vi "Test.vi"() -> ()   [LabVIEW 2021]
panel:
  out "x-1":i32
  out "size(s)":i32[](array[numeric])
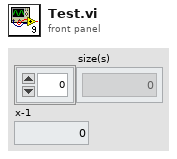
[diagram p1: front panel]
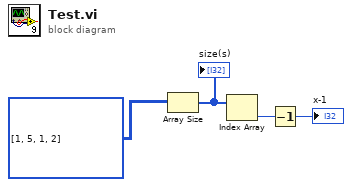
[diagram p0: block diagram]
diagram:
  n1 = Array Size(array=i32[][] [[1, 5, 1, 2]] ("Full array")) -> (size(s)=w4:i32[])
  "size(s)" <- w4
  n2 = Index Array(array=w4) -> (element=w3:i32)  [unwired: 1 in]
  n3 = Decrement(x=w3) -> (x-1=→"x-1":i32)
